vi "Decrease Gain.vi"(0 "System no.":i32=1 min=1 max=4 step=1, 1 "Board":i32=1 min=1 max=5 step=1, 2 "I(in)":dbl format="%.6f", 3 "Gain for I(in)":i32=10, 4 "Level":dbl=6.0 format="%.6f", 5 "error in":errorcluster) -> (14 "I (out)":dbl format="%.6f", 15 "Gain for I(out)":i32=10, 18 "Controller error":bool, 19 "error out":errorcluster)   [LabVIEW 2026]
doc: "Decreases gain if intensity is higher than Level."
panel:
  # "Decreases gain if intensity is higher than Level."
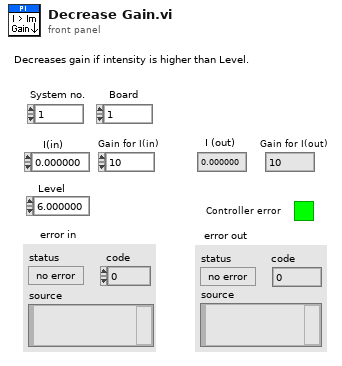
[diagram p1: front panel]
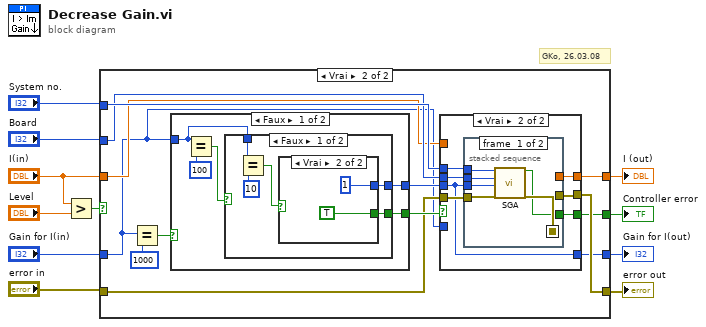
[diagram p0: block diagram]
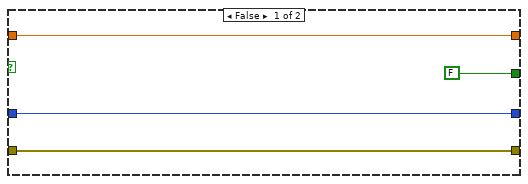
[diagram p2: hidden frame]
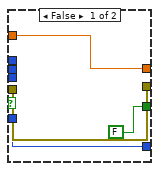
[diagram p3: hidden frame]
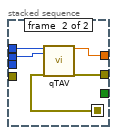
[diagram p4: hidden frame]
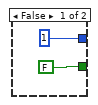
[diagram p5: hidden frame]
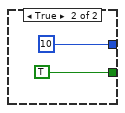
[diagram p6: hidden frame]
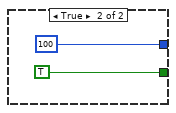
[diagram p7: hidden frame]
diagram:
  # "GKo, 26.03.08"
  n1 = Greater?(x="I(in)", y="Level") -> (0:w10:bool)
  n2 = case shown="Vrai" w10 {
    tunnel: "Gain for I(in)" -> [w13 w17]
    tunnel: "System no." -> [_ w25]
    tunnel: "Board" -> [_ w24]
    tunnel: "error in" -> [w15 w22]
    tunnel: [w15 w21] -> w2
    tunnel: [w14 w20] -> w6
    tunnel: "I(in)" -> [w14 w19]
    tunnel: [w13 w18] -> w4
    tunnel: [FALSE ("Controller error") w16] -> w1
    frame False {
    }
    frame True {
      n3 = Equal?(x=w17, y=1000) -> (x = y?=w27:bool)
      n4 = case shown="Faux" w27 {
        tunnel: [w53 100 ("y")] -> w23
        tunnel: w17 -> [w52 _]
        tunnel: [w51 TRUE] -> w26
        frame False {
          n5 = Equal?(x=w52, y=100) -> (x = y?=w54:bool)
          n6 = case shown="Faux" w54 {
            tunnel: [w57 10 ("y")] -> w53
            tunnel: w52 -> [w59 _]
            tunnel: [w56 TRUE] -> w51
            frame False {
              n7 = Equal?(x=w59, y=10) -> (x = y?=w58:bool)
              n8 = case shown="Vrai" w58 {
                tunnel: [1 ("y") 1 ("y")] -> w57
                tunnel: [FALSE TRUE] -> w56
                frame False {
                }
                frame True {
                }
              }
            }
            frame True {
            }
          }
        }
        frame True {
        }
      }
      n9 = case shown="Vrai" w26 {
        tunnel: w25 -> [_ w39]
        tunnel: w24 -> [_ w38]
        tunnel: w23 -> [_ w34]
        tunnel: w22 -> [w32 w37]
        tunnel: [w32 w36] -> w21
        tunnel: [w31 w35] -> w20
        tunnel: w19 -> [w31 _]
        tunnel: [w30 w34] -> w18
        tunnel: w17 -> [w30 _]
        tunnel: [FALSE ("Controller error") w33] -> w16
        frame False {
        }
        frame True {
          n10 = stacked-sequence {
            seq-local: [w41 _] -> [_ w50]
            tunnel: w39 -> [w45 w46]
            tunnel: w38 -> [w44 w47]
            tunnel: w34 -> [w43 _]
            tunnel: w37 -> [w42 _]
            tunnel: [_ w49] -> w36
            tunnel: [_ w48] -> w35
            tunnel: [w40 _] -> w33
            frame #0 {
              n11 = call "SGA.vi"("System no."=w45, "Board"=w44, "Gain"=w43, "error in"=w42) -> ("Controller error"=w40:bool, "error out"=w41:errorcluster)  [unwired: 14 out]
            }
            frame #1 {
              n12 = call "qTAV.vi"("System no."=w46, "Board"=w47, "error in"=w50) -> ("Analog value"=w48:dbl, "error out"=w49:errorcluster)  [unwired: 1 in, 14 out]
            }
          }
        }
      }
    }
  }
  "I (out)" <- w6
  "Gain for I(out)" <- w4
  "error out" <- w2
  "Controller error" <- w1
